vi "runtime test.vi"() -> ()   [LabVIEW 2013, in "async tests.lvlib"]
uses:
  async tests.lvlib
  configuration/asynchronous execution module configuration.lvclass
  runtime/asynchronous execution module runtime.lvclass
  tests/test module/module/execution/TEST RUNTIME.lvclass
  tests/test module/module/configuration/TEST CONFIGURATION.lvclass
  tests/test module/module/configuration/TEST CONFIGURATION.lvclass/TEST CONFIGURATION.ctl
  configuration/asynchronous execution module configuration.lvclass/asynchronous execution module configuration.ctl
  <vilib>/NI/Tag Bus/tag/tag descriptor.lvclass/tag descriptor.ctl
  <vilib>/NI/Tag Bus/dictionary/data dictionary.lvclass/data dictionary.ctl
  <vilib>/NI/Tag Bus/dictionary/lookup polymorphs/locate double.vi
  <vilib>/NI/Tag Bus/table/data polymorphs/write one/write Double.vi
  <vilib>/NI/Tag Bus/tag/read tag name.vi
  tests/test module/module/configuration/Read state module configuration.vi
  tests/test module/module/configuration/Read control functions.vi
  configuration/Write contained configuration.vi
  configuration/Write execution period (ms).vi
  <vilib>/NI/Tag Bus/dictionary/search/find data index.vi
  <vilib>/NI/Tag Bus/dictionary/search/search string list.vi
  <vilib>/NI/Tag Bus/dictionary/tag not found.vi
  <vilib>/NI/Tag Bus Module Framework/channel/TBM channel.lvclass
  <vilib>/NI/Tag Bus/dictionary/data dictionary.lvclass
  <vilib>/NI/Tag Bus/table/data table.lvlib
panel:
  in  "abort":bool
  out "result ok":bool
  out "param alloc ok":bool
  out "no error async":errorcluster
  out "exec settings ok":bool
  out "data alloc ok":bool
  out "results set":bool
  out "no error":errorcluster
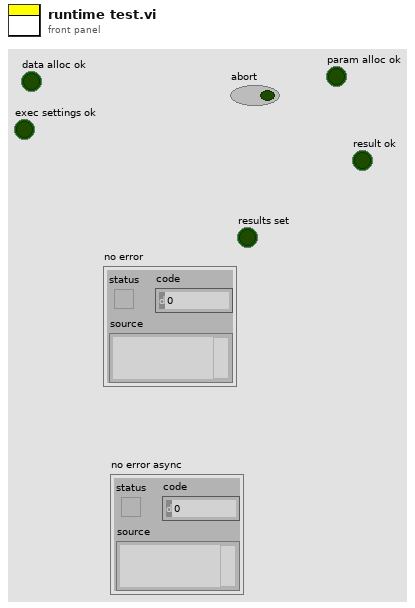
[diagram p1: front panel]
types:
  T1 = typedef "configuration tests.lvlib/TEST CONFIGURATION.lvclass/state module configuration.ctl" = cluster{"fixed input":refnum<class "TBM channel.lvclass">, "fixed output":refnum<class "TBM channel.lvclass">, "initial state":u8}
  T2 = typedef "configuration tests.lvlib/TEST CONFIGURATION.lvclass/control module configuration.ctl" = cluster{"name":string, "setpoint":refnum<class "TBM channel.lvclass">, "process variable":refnum<class "TBM channel.lvclass">, "output":refnum<class "TBM channel.lvclass">, "gains":T3, "output range":cluster{"output high":dbl, "output low":dbl}}
  T3 = typedef "configuration tests.lvlib/TEST CONFIGURATION.lvclass/gains.ctl" = cluster{"Kp":dbl, "Ki":dbl, "Kd":dbl}
  T4 = typedef "TBM channel.lvclass/data tables.ctl" = cluster{"input data":T5, "processing parameter":T5, "processing result":T5, "output data":T5}
  T5 = typedef "tag bus.lvlib/dictionary table pair.ctl" = cluster{"data dictionary":refnum<class "data dictionary.lvclass">, "data table":T6}
  T6 = typedef "tag bus.lvlib/data table.lvlib/data table.ctl" = cluster{"Double":dbl[], "Single":sgl[], "I64":i64[], "I32":i32[], "I16":i16[], "I8":i8[], "U64":u64[], "U32":u32[], "U16":u16[], "U8":u8[], "Boolean":bool[], "String":string[], "Array of Double":cluster{"DBL Array":dbl[]}[], "Array of Single":cluster{"SGL Array":sgl[]}[], "Array of I64":cluster{"I64 Array":i64[]}[], "Array of I32":cluster{"I32 Array":i32[]}[], "Array of I16":cluster{"I16 Array":i16[]}[], "Array of I8":cluster{"I8 Array":i8[]}[], "Array of U64":cluster{"U64 Array":u64[]}[], "Array of U32":cluster{"U32 Array":u32[]}[], "Array of U16":cluster{"U16 Array":u16[]}[], "Array of U8":cluster{"U8 Array":u8[]}[], "Array of Boolean":cluster{"Boolean Array":bool[]}[], "Array of String":cluster{"String Array":string[]}[]}
  T7 = typedef "TBM module execution interface.lvclass/execution settings.ctl" = cluster{"reads inputs":bool, "processes data":bool, "writes outputs":bool}
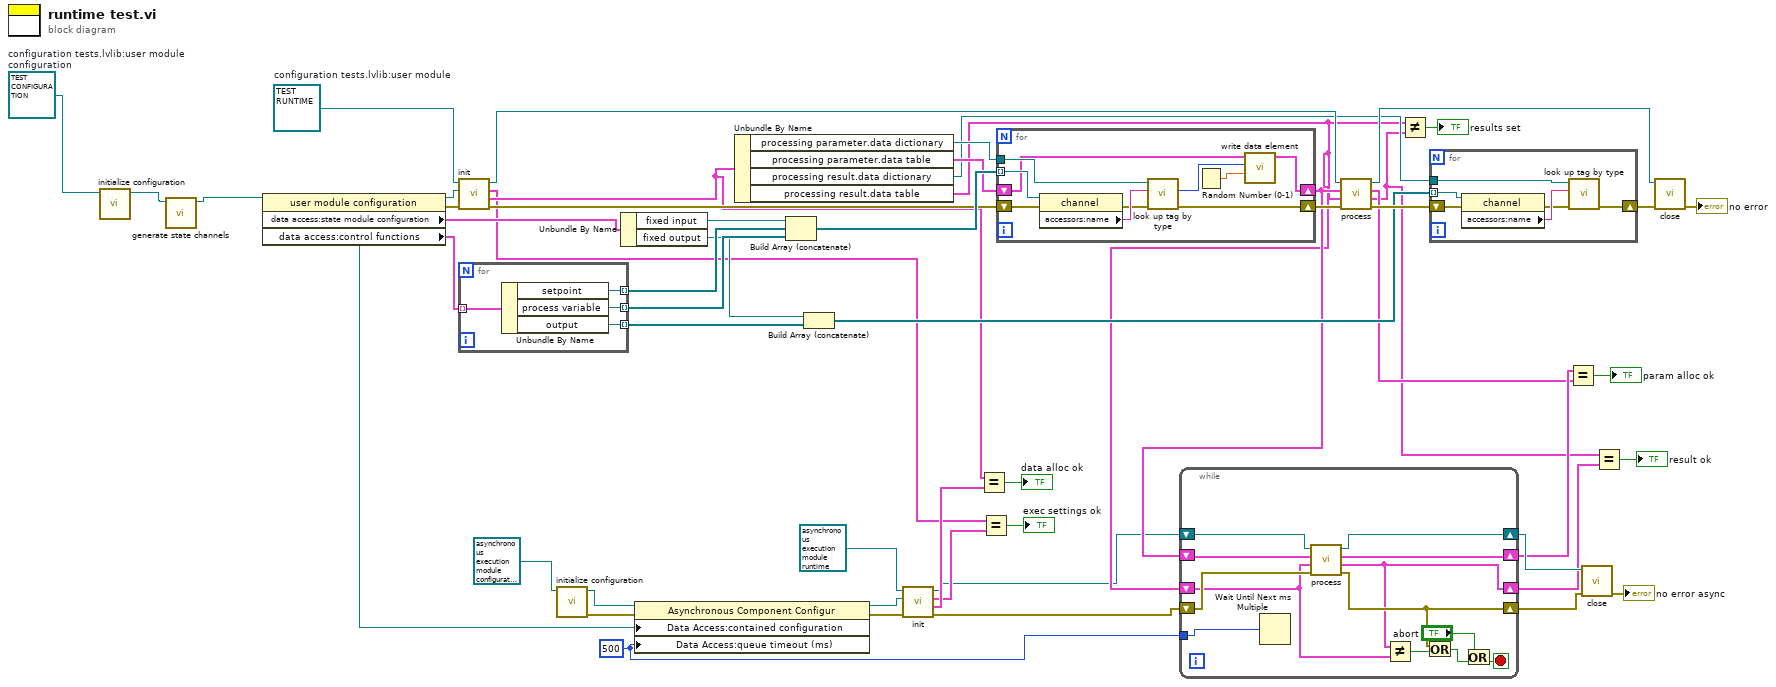
[diagram p0: block diagram]
diagram:
  w3 = refnum<class "TEST CONFIGURATION.lvclass"> refnum  # configuration tests.lvlib:user module configuration
  w4 = refnum<class "TEST RUNTIME.lvclass"> refnum  # configuration tests.lvlib:user module
  w18 = 500 ("queue timeout (ms)")
  n1 = call-dynamic "initialize configuration.vi"("configuration in"=w3) -> ("configuration out"=w2:refnum<class "TEST CONFIGURATION.lvclass">)  [unwired: 8 in, 2 out]
  n2 = call "generate state channels.vi"("tag bus configurable plugin module configuration in"=w2) -> ("tag bus configurable plugin module configuration out"=w1:refnum<class "TEST CONFIGURATION.lvclass">)  [unwired: 9 in, 1 out]
  n3 = property class="user module configuration"(reference=w1) -> (reference out=w50:refnum<class "TEST CONFIGURATION.lvclass">, error out=w51:errorcluster, "data access:state module configuration"=w49:T1, "data access:control functions"=w47:T2[])  [unwired: 1 in]
  n4 = call-dynamic "init.vi"("error in"=w51, "TBM module configuration in"=w50, "tag bus configurable plugin module in"=w4) -> ("error out"=w38:errorcluster, "data allocations"=w24:T4, "execution settings"=w22:T7, "tag bus configurable plugin module out"=w48:refnum<class "TEST RUNTIME.lvclass">)  [unwired: 5 in]
  n5 = for {
    tunnel: w47 -> [w56] mode=indexing
    tunnel: [w55] -> w45 mode=indexing
    tunnel: [w54] -> w44 mode=indexing
    tunnel: [w53] -> w43 mode=indexing
    n6 = Unbundle By Name(w56) -> ("setpoint"=w55:refnum<class "TBM channel.lvclass">, "process variable"=w54:refnum<class "TBM channel.lvclass">, "output"=w53:refnum<class "TBM channel.lvclass">)
  }
  n7 = call-dynamic "initialize configuration.vi"("configuration in"=refnum<class "asynchronous execution module configuration.lvclass"> refnum ("Asynchronous Component Configuration")) -> ("error out"=w28:errorcluster, "configuration out"=w29:refnum<class "asynchronous execution module configuration.lvclass">)  [unwired: 8 in, 1 out]
  n8 = Unbundle By Name(w49) -> ("fixed input"=w46:refnum<class "TBM channel.lvclass">, "fixed output"=w42:refnum<class "TBM channel.lvclass">)
  n9 = property class="Asynchronous Component Configur"(reference=w29, error in=w28, "Data Access:contained configuration"=w1, "Data Access:queue timeout (ms)"=w18) -> (reference out=w26:refnum<class "asynchronous execution module configuration.lvclass">, error out=w27:errorcluster)
  n10 = Unbundle By Name(w24) -> ("processing parameter.data dictionary"=w41:refnum<class "data dictionary.lvclass">, "processing parameter.data table"=w37:T6, "processing result.data dictionary"=w31:refnum<class "data dictionary.lvclass">, "processing result.data table"=w16:T6)
  n11 = Build Array (concatenate)(w46, w45, w44) -> (w40:refnum<class "TBM channel.lvclass">[])
  n12 = Build Array (concatenate)(w42, w43) -> (w32:refnum<class "TBM channel.lvclass">[])
  n13 = call-dynamic "init.vi"("error in"=w27, "component configuration"=w26, "asynchronous execution module runtime In"=refnum<class "asynchronous execution module runtime.lvclass"> refnum ("Asynchronous Component Runtime")) -> ("error out"=w14:errorcluster, "data allocations"=w23:T4, "execution settings"=w21:T7, "asynchronous execution module runtime Out"=w15:refnum<class "asynchronous execution module runtime.lvclass">)  [unwired: 5 in]
  n14 = Equal?(x=w24, y=w23) -> (x = y?=→"data alloc ok":bool)
  n15 = Equal?(x=w22, y=w21) -> (x = y?=→"exec settings ok":bool)
  n16 = for {
    tunnel: w41 -> [w66]
    tunnel: w40 -> [w65] mode=indexing
    shift-right: [w62] -> w39
    shift-left: w38 -> [w61]
    shift-right: [w59] -> w17
    shift-left: w37 -> [w60]
    n17 = property class="channel"(reference=w65, error in=w61) -> (error out=w63:errorcluster, "accessors:name"=w64:string)  [unwired: 1 out]
    n18 = call-poly <vilib>:"look up tag by type.vi"("error in"=w63, "name"=w64, "data dictionary in"=w66) -> ("error out"=w62:errorcluster, "index"=w58:i32)  [unwired: 6 in, 1 out]
    n19 = Random Number (0-1)() -> (number: 0 to 1=w57:dbl)
    n20 = call-poly <vilib>:"write data element.vi"("value"=w57, "index"=w58, "data table in"=w60) -> ("data table out"=w59:T6)  [unwired: 8 in]
  }
  n21 = while {
    tunnel: w18 -> [w79]
    shift-right: [w69] -> w10
    shift-left: w17 -> [w70]
    shift-right: [w72] -> w5
    shift-left: w16 -> [w71]
    shift-right: [w78] -> w12
    shift-left: w15 -> [w77]
    shift-right: [w74] -> w11
    shift-left: w14 -> [w76]
    stop <- w68 stop-if-true
    n22 = Wait Until Next ms Multiple(millisecond multiple=w79) -> ()  [unwired: 1 out]
    n23 = call-dynamic "process.vi"("error in"=w76, "result allocation"=w71, "data to process"=w70, "module in"=w77) -> ("error out"=w74:errorcluster, "result data"=w72:T6, "processing allocation"=w69:T6, "module out"=w78:refnum<class "asynchronous execution module runtime.lvclass">)  [unwired: 4 in]
    n24 = Not Equal?(x=w72, y=w71) -> (x != y?=w75:bool)
    n25 = Or(x=w74, y=w75) -> (x .or. y?=w73:bool)
    n26 = Or(x="abort", y=w73) -> (x .or. y?=w68:bool)
  }
  n27 = call-dynamic "process.vi"("error in"=w39, "result allocation"=w16, "parameters"=w17, "module in"=w48) -> ("error out"=w35:errorcluster, "results"=w6:T6, "parameter allocation"=w9:T6, "module out"=w36:refnum<class "TEST RUNTIME.lvclass">)  [unwired: 4 in]
  n28 = Not Equal?(x=w16, y=w6) -> (x != y?=→"results set":bool)
  n29 = for {
    tunnel: w32 -> [w85] mode=indexing
    shift-right: [w82] -> w34
    shift-left: w35 -> [w81]
    tunnel: w31 -> [w80]
    n30 = property class="channel"(reference=w85, error in=w81) -> (error out=w83:errorcluster, "accessors:name"=w84:string)  [unwired: 1 out]
    n31 = call-poly <vilib>:"look up tag by type.vi"("error in"=w83, "name"=w84, "data dictionary in"=w80) -> ("error out"=w82:errorcluster)  [unwired: 6 in, 2 out]
  }
  n32 = Equal?(x=w10, y=w9) -> (x = y?=→"param alloc ok":bool)
  n33 = call-dynamic "close.vi"("error in"=w11, "asynchronous execution module runtime In"=w12) -> ("error out"=→"no error async":errorcluster)  [unwired: 9 in]
  n34 = Equal?(x=w6, y=w5) -> (x = y?=→"result ok":bool)
  n35 = call-dynamic "close.vi"("error in"=w34, "tag bus configurable plugin module in"=w36) -> ("error out"=→"no error":errorcluster)  [unwired: 9 in]
